vi "Graph Annotations.vi"() -> ()   [LabVIEW 2023]
doc: "This example demonstrates how to programmatically change the values of annotations. A random plot is generated. The average, minimum, and maximum values of the plot are calculated and annotated."
panel:
  in  "Average":string="Average = "
  out "Waveform Graph":dbl[](graph)
  # "Overview: Demonstrates the use of Graph Annotations to display textual information within a graph.\nInstructions:\nRun the VI. Annotations will appear within the graph identifying the maximum, minimum, and average values of the data. See the block diagram for more information."
  # "To create a new annotation on a graph, right-click the graph and select Data Operations > Create Annotation."
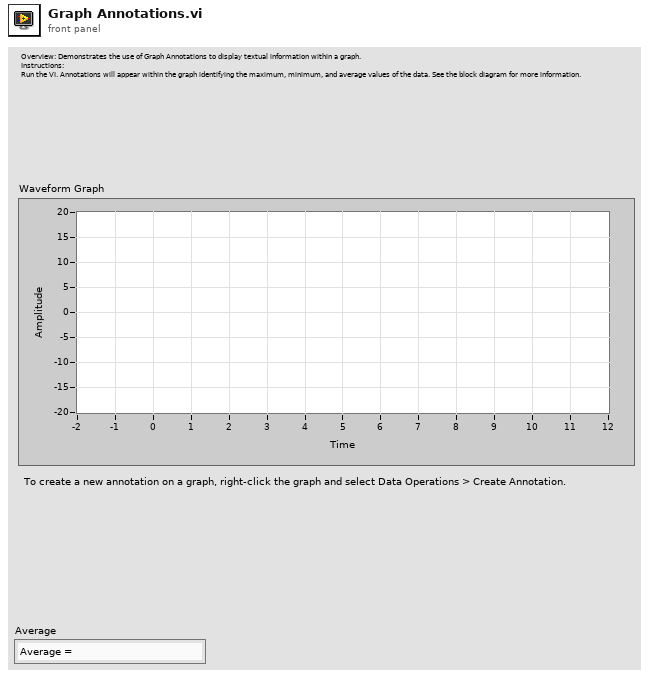
[diagram p1: front panel]
types:
  T1 = typedef "LVAnnotationListTypeDef.ctl" = cluster{"Name":string, "Color":u32, "Style":u8, "Point Style":u8, "Name Visible":bool, "Allow Drag":bool, "Annotation Mode":u32, "Plot":i32, "Index":i32, "Position":cluster{"X":dbl, "Y":dbl}, "X Scale":u32, "Y Scale":u32, "Show Arrow":bool, "Lock Name":bool, "Plot Area":i32, "Label Offset":cluster{"X":dbl, "Y":dbl}}[]
  T2 = cluster{"Name":string, "Color":u32, "Style":u8, "Point Style":u8, "Name Visible":bool, "Allow Drag":bool, "Annotation Mode":u32, "Plot":i32, "Index":i32, "Position":cluster{"X":dbl, "Y":dbl}, "X Scale":u32, "Y Scale":u32, "Show Arrow":bool, "Lock Name":bool, "Plot Area":i32, "Label Offset":cluster{"X":dbl, "Y":dbl}}
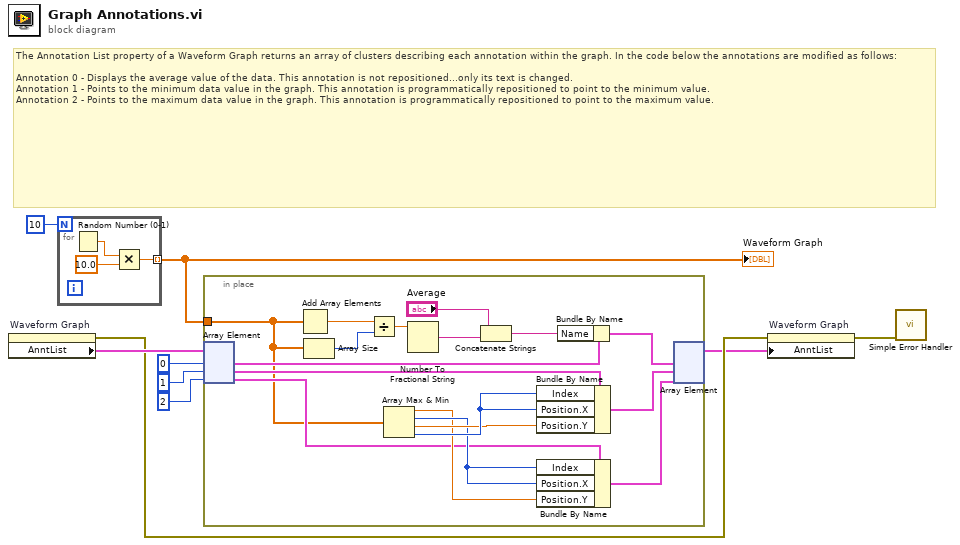
[diagram p0: block diagram]
diagram:
  # "The Annotation List property of a Waveform Graph returns an array of clusters describing each annotation within the graph. In the code below the annotations are modified as follows:\n\nAnnotation 0 - Displays the average value of the data. This annotation is not repositioned...only its text is changed.\nAnnotation 1 - Points to the minimum data value in the graph. This annotation is programmatically repositioned to point to the minimum value.\nAnnotation 2 - Points to the maximum data value in the graph. This annotation is programmatically repositioned to point to the maximum value."
  n1 = property on="Waveform Graph" class="WaveformGraph (strict)"() -> (error out=w3:errorcluster, "AnntList"=w8:T1)  [unwired: 2 in, 1 out]
  n2 = for {
    N: 10 -> [_]
    tunnel: [w10] -> w4 mode=indexing
    n3 = Random Number (0-1)() -> (number: 0 to 1=w12:dbl)
    n4 = Multiply(x=w12, y=10.0) -> (x*y=w10:dbl)
  }
  "Waveform Graph" <- w4
  n5 = in-place {
    in-place-border: w4 -> [w14]
    n6 = in-place-array #1(w8, 0, 1, 2) -> (w25:T2, w21:T2, w16:T2)
    n7 = Add Array Elements(numeric array=w14) -> (sum=w15:dbl)
    n8 = Array Size(array=w14) -> (size(s)=w13:i32)
    n9 = Divide(x=w15, y=w13) -> (x/y=w29:dbl)
    n10 = Array Max & Min(array=w14) -> (max value=w18:dbl, max index (indices)=w19:i32, min value=w22:dbl, min index (indices)=w23:i32)
    n11 = Number To Fractional String(number=w29) -> (F-format string=w27:string)  [unwired: 3 in]
    n12 = Concatenate Strings("Average", w27) -> (w26:string)
    n13 = Bundle By Name(cluster=w21, "Index"=w23, "Position.X"=w23, "Position.Y"=w22) -> (w20:T2)
    n14 = Bundle By Name(cluster=w16, "Index"=w19, "Position.X"=w19, "Position.Y"=w18) -> (w17:T2)
    n15 = Bundle By Name(cluster=w25, "Name"=w26) -> (w24:T2)
    n16 = in-place-array #1(w24, w20, w17) -> (w1:T1)  [unwired: 3 out]
  }
  n17 = property on="Waveform Graph" class="WaveformGraph (strict)"(error in=w3, "AnntList"=w1) -> (error out=w2:errorcluster)  [unwired: 1 in, 1 out]
  n18 = call <vilib>:"Simple Error Handler.vi"("error in (no error)"=w2) -> ()  [unwired: 4 in, 5 out]
